vi "Random VI Example.vi"() -> ()   [LabVIEW 2011]
uses:
  <vilib>/rvi/Analysis/measure/FFT/XNode/niFpgaFFT.xnode
  <vilib>/rvi/Analysis/measure/FFT/XNode/niFpgaFFTButterflyDelays.ctl
  <vilib>/fxp/LVFixedPointQuantizationPolicyTypeDef.ctl
  <vilib>/rvi/Analysis/measure/FFT/simModelSupport/niFpgaFFTSimDfxp.ctl
  <vilib>/rvi/Analysis/measure/FFT/simModelSupport/niFpgaFFTSimArithmeticProperties.ctl
  <vilib>/rvi/Analysis/measure/FFT/simModelSupport/niFPGA FFT Sim Types.ctl
  <vilib>/rvi/Analysis/measure/FFT/simModelSupport/niFPGA FFT Sim Stream Group Properties.ctl
  <vilib>/rvi/Analysis/measure/FFT/simModelSupport/niFPGA FFT Streaming Sim Properties.ctl
  <vilib>/rvi/Analysis/measure/FFT/simModelSupport/niFpgaFFTSimModelStreamingCore.vi
panel:
  in  "reset":bool
  in  "N":u16
  in  "Input":bool
  out "Debounced Output":bool
  out "Debounced Output":bool
  in  "Input":bool
  out "Falling Edge":bool
  out "Rising Edge":bool
  out "Any Edge":bool
  in  "SCLK":bool
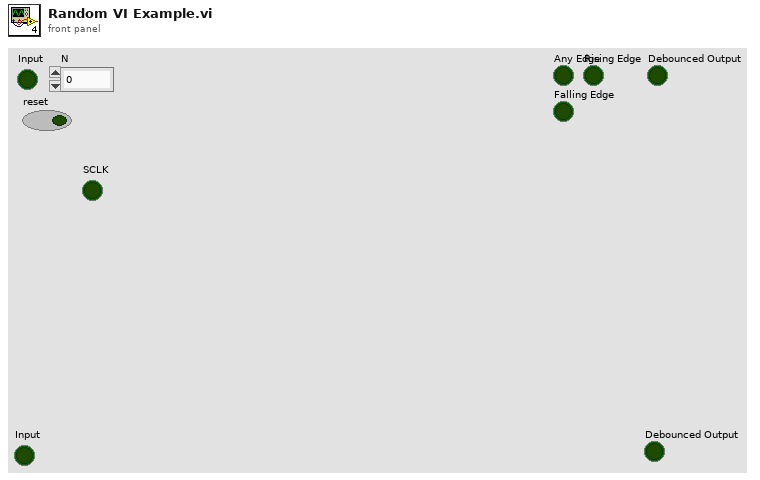
[diagram p1: front panel]
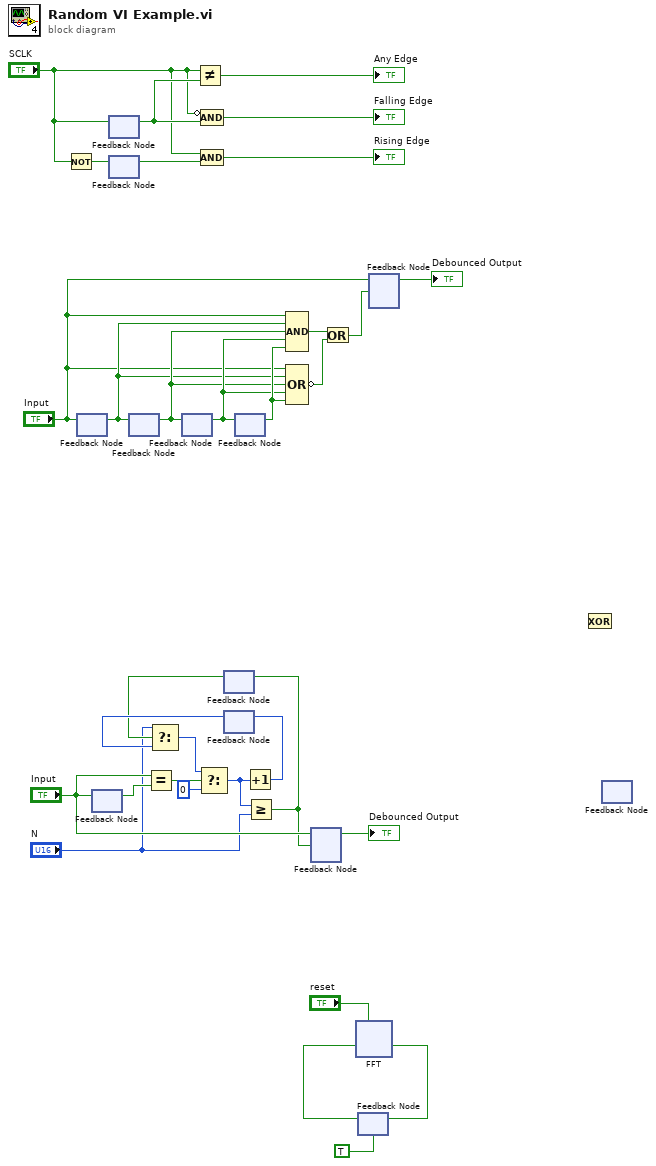
[diagram p0: block diagram]
diagram:
  n1 = Not(x="SCLK") -> (.not. x?=w32:bool)
  n2 = feedback #1() -> (w22:bool)  [unwired: 1 in]
  n3 = feedback-in #1("Input") -> ()
  n4 = feedback #2() -> (w16:bool)  [unwired: 1 in]
  n5 = feedback-in #2("Input") -> ()
  n6 = feedback-in #3("SCLK") -> ()
  n7 = feedback #3() -> (w28:bool)  [unwired: 1 in]
  n8 = feedback #4() -> (w31:bool)  [unwired: 1 in]
  n9 = feedback-in #4(w32) -> ()
  n10 = feedback #5() -> (w23:bool)  [unwired: 1 in]
  n11 = feedback-in #5(w22) -> ()
  n12 = Equal?(x="Input", y=w16) -> (x = y?=w15:bool)
  n13 = feedback #6() -> (w24:bool)  [unwired: 1 in]
  n14 = feedback-in #6(w23) -> ()
  n15 = Not Equal?(x="SCLK", y=w28) -> (x != y?=→"Any Edge":bool)
  n16 = Compound Arithmetic op=AND(invert "SCLK", w28) -> (→"Falling Edge":bool)
  n17 = Compound Arithmetic op=AND("SCLK", w31) -> (→"Rising Edge":bool)
  n18 = feedback #7() -> (w6:bool)  [unwired: 1 in]
  n19 = feedback #8() -> (w9:u16)  [unwired: 1 in]
  n20 = Select(t="N", s=w6, f=w9) -> (s? t:f=w8:u16)
  n21 = Select(t=w8, s=w15, f=u16 0) -> (s? t:f=w11:u16)
  n22 = feedback #9() -> (w25:bool)  [unwired: 1 in]
  n23 = feedback-in #9(w24) -> ()
  n24 = Increment(x=w11) -> (x+1=w14:u16)
  n25 = feedback-in #8(w14) -> ()
  n26 = Greater Or Equal?(x=w11, y="N") -> (x >= y?=w7:bool)
  n27 = feedback-in #7(w7) -> ()
  n28 = Compound Arithmetic op=AND("Input", w22, w23, w24, w25) -> (w21:bool)
  n29 = Compound Arithmetic op=OR("Input", w22, w23, w24, w25) -> (invert w20:bool)
  n30 = feedback #10() -> (→"Debounced Output":bool)  [unwired: 1 in]
  n31 = feedback-in #10("Input", w7) -> ()
  n32 = Or(x=w21, y=w20) -> (x .or. y?=w18:bool)
  n33 = feedback #11(TRUE ("output valid")) -> (w2:bool)
  n34 = xnode "FFT"("reset"="reset", "input valid"=w2) -> ("output valid"=w3:bool)  [unwired: 3 in, 4 out]
  n35 = feedback-in #11(w3) -> ()
  n36 = feedback #12() -> (→"Debounced Output":bool)  [unwired: 1 in]
  n37 = feedback-in #12("Input", w18) -> ()
  n38 = Exclusive Or() -> ()  [unwired: 2 in, 1 out]
  n39 = feedback #13() -> ()  [unwired: 2 in]
  n40 = feedback-in #13() -> ()  [unwired: 1 out]
